vi "FTW-Actor-Log-FrameworkEvent.vi"(0 "FTW Actor Instance":refnum<class "FTW-ActorInstance.lvclass">, 5 "Framework Event":T1, 7 "Event Data":string, 11 "error in":errorcluster) -> (4 "FTW Actor Instance out":refnum<class "FTW-ActorInstance.lvclass">, 15 "error out":errorcluster)   [LabVIEW 2013, in "FTW-ActorInstance.lvclass"]
uses:
  FTW-ActorInstance.lvclass
  FTW-Actor-FrameworkEvent.ctl
panel:
  # "Inputs"
  # "Outputs"
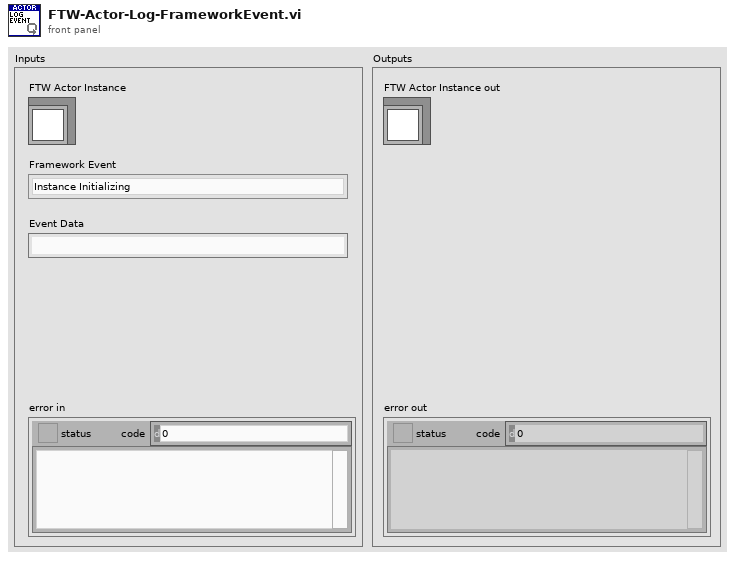
[diagram p1: front panel]
types:
  T1 = typedef "FTW-ActorInstance.lvclass/FTW-Actor-FrameworkEvent.ctl" = enum16{"Instance Initializing", "Instance Constructed", "Instance Initialized", "Instance Job", "Instance Handle Request", "Instance Shutting Down", "Instance Destroyed"}
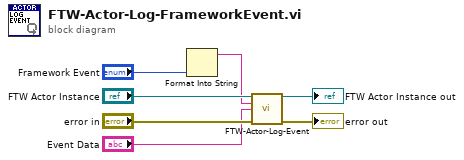
[diagram p0: block diagram]
diagram:
  n1 = Format Into String("Framework Event") -> (resulting string=w1:string)  [unwired: 3 in, 1 out]
  n2 = call-dynamic "FTW-Actor-Log-Event.vi"("FTW Actor Instance"="FTW Actor Instance", "Event Type"=w1, "Event Data"="Event Data", "error in"="error in") -> ("FTW Actor Instance out"=→"FTW Actor Instance out":refnum<class "FTW-ActorInstance.lvclass">, "error out"=→"error out":errorcluster)  [unwired: 9 in, 1 out]
